vi "Larger_Smaller_Determiner.vi"(1 "Input B":dbl, 2 "Get Flag":enum16{"LARGER", "SMALLER"}(ring), 3 "Input A":dbl) -> (0 "Output Number":dbl)   [LabVIEW 2016]
doc: "Help by FRC Team 836 - The RoboBees\n\nThis VI takes two numbers and returns the \"Larger\" or \"Smaller\" number \ndepending on the \"Get Flag\" setting."
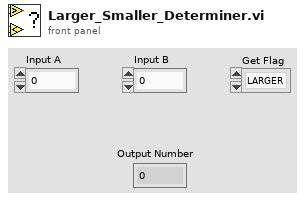
[diagram p1: front panel]
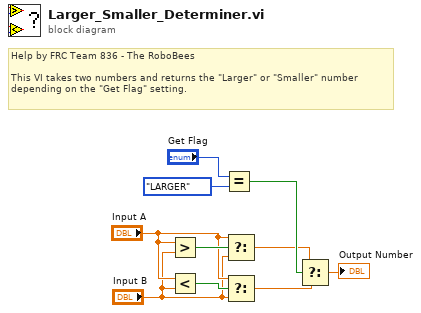
[diagram p0: block diagram]
diagram:
  # "Help by FRC Team 836 - The RoboBees\n\nThis VI takes two numbers and returns the \"Larger\" or \"Smaller\" number \ndepending on the \"Get Flag\" setting."
  n1 = Greater?(x="Input A", y="Input B") -> (0:w10:bool)
  n2 = Less?(x="Input A", y="Input B") -> (x < y?=w9:bool)
  n3 = Equal?(x="Get Flag", y=enum16{"LARGER", "SMALLER"}."LARGER") -> (x = y?=w5:bool)
  n4 = Select(t="Input A", s=w10, f="Input B") -> (s? t:f=w2:dbl)
  n5 = Select(t="Input A", s=w9, f="Input B") -> (s? t:f=w1:dbl)
  n6 = Select(t=w2, s=w5, f=w1) -> (s? t:f=→"Output Number":dbl)
